vi "test.vi"() -> ()   [LabVIEW 2020]
uses:
  <vilib>/userdefined/High Color/IMAQdx.ctl
  <vilib>/vision/NI_Vision_Development_Module.lvlib
  <vilib>/vision/driver/NI_Vision_Acquisition_Software.lvlib
panel:
  out "Array":string[](array[string])
  out "error out":errorcluster
  out "Number of Particles":i32
  in  "Window Size (32x32)":cluster{"SizeX":i32, "SizeY":i32}={"SizeX"=32, "SizeY"=32} {"SizeY" min=3 step=1; "SizeX" min=3 step=1}
  in  "Selection Values":T2(array[cluster]) {"Measurement Parameter" items=["Center of Mass X", "Center of Mass Y", "First Pixel X", "First Pixel Y", "Bounding Rect Left", "Bounding Rect Top", "Bounding Rect Right", "Bounding Rect Bottom", "Max Feret Diameter Start X", "Max Feret Diameter Start Y", "Max Feret Diameter End X", "Max Feret Diameter End Y", "Max Horiz. Segment Length Left", "Max Horiz. Segment Length Right", "Max Horiz. Segment Length Row", "-", "Bounding Rect Width", "Bounding Rect Height", "Bounding Rect Diagonal", "Perimeter", "Convex Hull Perimeter", "Holes' Perimeter", "Max Feret Diameter", "Equivalent Ellipse Major Axis", "Equivalent Ellipse Minor Axis", "Equivalent Ellipse Minor Axis (Feret)", "Equivalent Rect Long Side", "Equivalent Rect Short Side", "Equivalent Rect Diagonal", "Equivalent Rect Short Side (Feret)", "Average Horiz. Segment Length", "Average Vert. Segment Length", "Hydraulic Radius", "Waddel Disk Diameter", "-", "Area", "Holes' Area", "Particle & Holes' Area", "Convex Hull Area", "Image Area", "-", "Number of Holes", "Number of Horiz. Segments", "Number of Vert. Segments", "-", "Orientation", "Max Feret Diameter Orientation", "-", "% Area/Image Area", "% Area/(Particle & Holes' Area)", "Ratio of Equivalent Ellipse Axes", "Ratio of Equivalent Rect Sides", "-", "Elongation Factor", "Compactness Factor", "Heywood Circularity Factor", "Type Factor", "-", "Sum X", "Sum Y", "Sum XX", "Sum XY", "Sum YY", "Sum XXX", "Sum XXY", "Sum XYY", "Sum YYY", "-", "Moment of Inertia XX", "Moment of Inertia XY", "Moment of Inertia YY", "Moment of Inertia XXX", "Moment of Inertia XXY", "Moment of Inertia XYY", "Moment of Inertia YYY", "Norm. Moment of Inertia XX", "Norm. Moment of Inertia XY", "Norm. Moment of Inertia YY", "Norm. Moment of Inertia XXX", "Norm. Moment of Inertia XXY", "Norm. Moment of Inertia XYY", "Norm. Moment of Inertia YYY", "Hu Moment 1", "Hu Moment 2", "Hu Moment 3", "Hu Moment 4", "Hu Moment 5", "Hu Moment 6", "Hu Moment 7"]; "Range Lower Value" format="%.2f"; "Range Upper Value" format="%.2f"}
  in  "Look For (Bright Objects)":u32(ring) items=["Bright Objects", "Dark Objects"]
  out "Image":T3(plugin-control)
  in  "stop threshold":bool
  in  "start":bool
  in  "Calibrazione":bool
  out "Input Image 1":T3(plugin-control)
  in  "Stop Acquisizione":bool
  out "Array of Real World Coordinates":cluster{"X":sgl, "Y":sgl}[](array[cluster]) {"Y" format="%.2f"; "X" format="%.2f"}
  in  "error in (no error)":errorcluster
  in  "Session In":T4="cam1"
  in  "Dove salvo l'immagine Calib Info":path=path "C:/Users/Dell/Documents/Vision-Systems/calib-info.png"
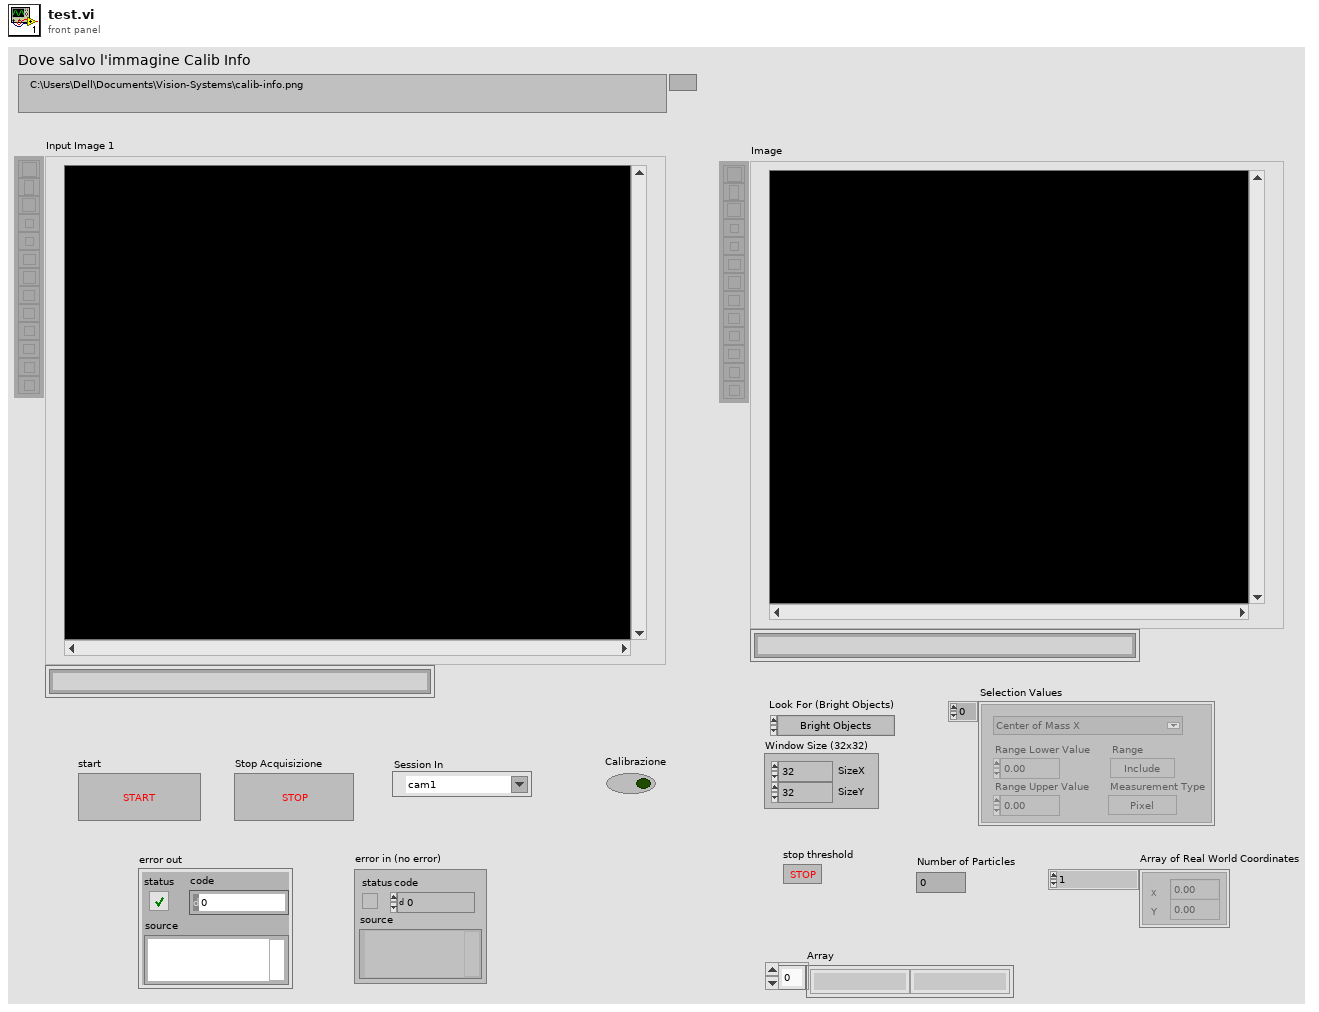
[diagram p1: front panel]
types:
  T1 = typedef "Particle Parameters" = i32
  T2 = cluster{"Measurement Parameter":T1, "Range Lower Value":dbl, "Range Upper Value":dbl, "Range":bool, "Measurement Type":bool}[]
  T3 = typedef "IMAQ Image.ctl" = refnum<image>
  T4 = typedef "IMAQdx.ctl" = refnum<k21>
  T5 = cluster{"Origin Pixel":cluster{"X":sgl, "Y":sgl}, "Angle Relative to Horizontal (deg)":sgl, "Axis Reference":u32}
  T6 = cluster{"Origin Pixel":cluster{"X":sgl, "Y":sgl}, "Angle Relative to Horizontal (deg)":sgl, "X Axis Pixel":cluster{"X":sgl, "Y":sgl}, "Axis Reference":u32}
  T7 = typedef "Image Type" = u32
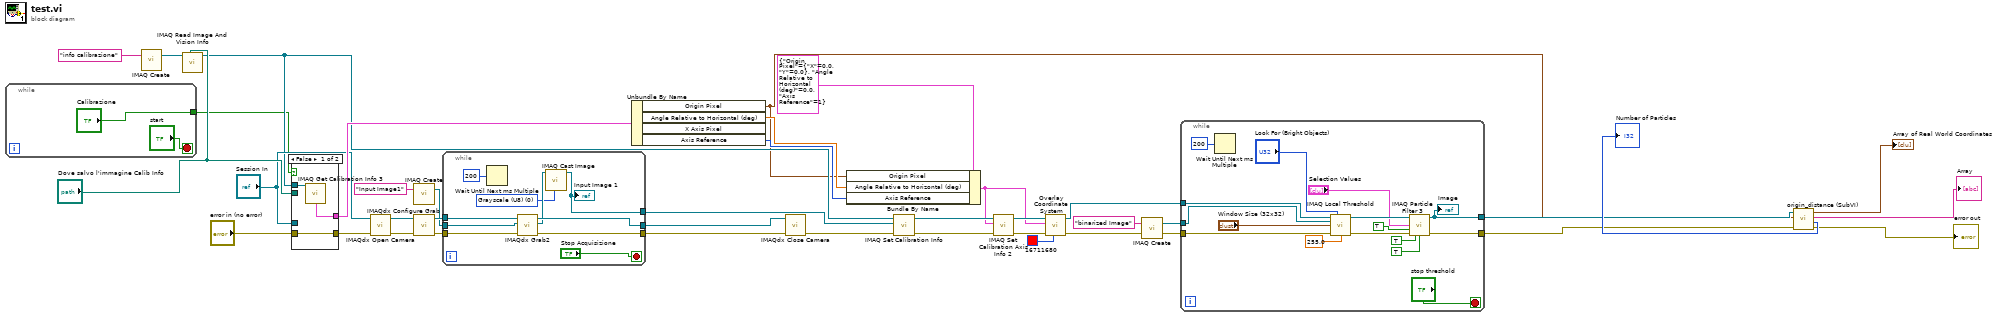
[diagram p0: block diagram]
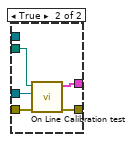
[diagram p2: hidden frame]
diagram:
  n1 = while {
    tunnel: ["Calibrazione"] -> w15
    stop <- "start" stop-if-true
  }
  n2 = call "IMAQ Create"("Image Name"="info calibrazione") -> ("New Image"=w17:T3)  [unwired: 4 in, 1 out]
  n3 = call "IMAQ Read Image And Vision Info"("File Path"="Dove salvo l'immagine Calib Info", "Image"=w17) -> ("Image Out"=w16:T3)  [unwired: 7 in, 2 out]
  n4 = case shown="False" w15 {
    tunnel: "Dove salvo l'immagine Calib Info" -> [_ w50]
    tunnel: "error in (no error)" -> [w45 w49]
    tunnel: [w44 w48] -> w27
    tunnel: "Session In" -> [_ w47]
    tunnel: [w45 w46] -> w18
    tunnel: w16 -> [w43 _]
    frame False {
      n5 = call "IMAQ Get Calibration Info 3"("Calibration Template Image"=w43) -> ("Calibration Axis Info"=w44:T6)  [unwired: 6 in, 8 out]
    }
    frame True {
      n6 = call "On Line Calibration test.vi"("error in (no error)"=w49, "Session In"=w47, "Dove salvo l'immagine Calib Info"=w50) -> ("error out"=w46:errorcluster, "Calibration Axis Info"=w48:T6)  [unwired: 7 in]
    }
  }
  n7 = call <vilib>:"IMAQdx Open Camera.vi"("error in"=w18, "Session In"="Session In") -> ("error out"=w24:errorcluster, "Session Out"=w25:T4)  [unwired: 8 in]
  n8 = call "IMAQ Create"("Image Name"="Input Image1") -> ("New Image"=w20:T3)  [unwired: 4 in, 1 out]
  n9 = call <vilib>:"IMAQdx Configure Grab.vi"("error in"=w24, "Session In"=w25) -> ("error out"=w23:errorcluster, "Session Out"=w26:T4)  [unwired: 8 in]
  n10 = while {
    tunnel: w26 -> [w58]
    tunnel: w23 -> [w57]
    tunnel: [w56] -> w22
    tunnel: [w55] -> w21
    tunnel: [w52] -> w14
    tunnel: w20 -> [w51]
    stop <- "Stop Acquisizione" stop-if-true
    w53 = T7 0 items=["Grayscale (U8)", "Grayscale (I16)", "Grayscale (SGL)", "Complex (CSG)", "RGB (U32)", "HSL (U32)", "RGB (U64)", "Grayscale (U16)"] ("Image Type")
    n11 = Wait Until Next ms Multiple(millisecond multiple=u32 200) -> ()  [unwired: 1 out]
    n12 = call <vilib>:"IMAQdx Grab2.vi"("error in"=w57, "Image In"=w51, "Session In"=w58) -> ("error out"=w55:errorcluster, "Image Out"=w54:T3, "Session Out"=w56:T4)  [unwired: 5 in, 1 out]
    n13 = call "IMAQ Cast Image"("Image Type"=w53, "Image Src"=w54) -> ("Image Dst Out"=w52:T3)  [unwired: 8 in, 1 out]
    "Input Image 1" <- w52
  }
  n14 = Unbundle By Name(w27) -> ("Origin Pixel"=w1:cluster{"X":sgl, "Y":sgl}, "Angle Relative to Horizontal (deg)"=w31:sgl, "Axis Reference"=w32:u32)  [unwired: 1 out]
  n15 = call <vilib>:"IMAQdx Close Camera.vi"("error in"=w21, "Session In"=w22) -> ("error out"=w8:errorcluster)  [unwired: 9 in]
  n16 = Bundle By Name(cluster=T5 {"Origin Pixel"={"X"=0.0, "Y"=0.0}, "Angle Relative to Horizontal (deg)"=0.0, "Axis Reference"=1} ("Calibration Axis Info"), "Origin Pixel"=w1, "Angle Relative to Horizontal (deg)"=w31, "Axis Reference"=w32) -> (w30:T5)
  n17 = call "IMAQ Set Calibration Info"("error in (no error)"=w8, "Image Dst"=w14, "Image Src"=w16) -> ("error out"=w37:errorcluster, "Calibrated Image"=w38:T3)  [unwired: 7 in]
  n18 = call-poly "IMAQ Set Calibration Axis Info 2"("error in (no error)"=w37, "Calibration Axis Info"=w30, "Calibration Template Image In"=w38) -> ("error out"=w35:errorcluster, "Calibration Template Image Out"=w36:T3)  [unwired: 7 in]
  n19 = call "Overlay Coordinate System.vi"("Color"=u32 16711680, "error in"=w35, "Calibration Axis Info"=w30, "Image"=w36) -> ("error out"=w10:errorcluster, "Image Out"=w13:T3)  [unwired: 6 in]
  n20 = call "IMAQ Create"("Image Name"="binarized Image", "error in (no error)"=w10) -> ("New Image"=w11:T3, "error out"=w9:errorcluster)  [unwired: 3 in]
  n21 = while {
    tunnel: [w73] -> w2
    tunnel: w13 -> [w76]
    tunnel: w11 -> [w70]
    tunnel: w9 -> [w63]
    tunnel: [w61] -> w3
    stop <- "stop threshold" stop-if-true
    n22 = Wait Until Next ms Multiple(millisecond multiple=u32 200) -> ()  [unwired: 1 out]
    n23 = call "IMAQ Local Threshold"("Image Src"=w76, "Look For (Bright Objects)"="Look For (Bright Objects)", "Image Dst"=w70, "Window Size (32x32)"="Window Size (32x32)", "error in (no error)"=w63, "Replace Value (1)"=sgl 255.0) -> ("Image Dst Out"=w72:T3, "error out"=w62:errorcluster)  [unwired: 8 in]
    n24 = call "IMAQ Particle Filter 3"("Image Src"=w72, "Selection Values"="Selection Values", "Keep/Remove Particles (F)"=TRUE, "error in (no error)"=w62, "Reject Border? (F)"=TRUE, "Fill Holes? (F)"=TRUE) -> ("Image Dst Out"=w73:T3, "error out"=w61:errorcluster)  [unwired: 7 in, 1 out]
    "Image" <- w73
  }
  n25 = call "origin_distance (SubVI).vi"("error in (no error)"=w3, "Origin Pixel"=w1, "Refnum in"=w2) -> ("error out"=→"error out":errorcluster, "Number of Particles"=→"Number of Particles":i32, "Array"=→"Array":string[], "Array of Real World Coordinates"=→"Array of Real World Coordinates":cluster{"X":sgl, "Y":sgl}[])  [unwired: 5 in]
